vi "index.vi"() -> ()   [LabVIEW 2023]
panel:
  in  "Blank":bool
  in  "label printing":bool
  in  "close call":bool
  in  "Report":bool
  in  "stop":bool
  in  "Vendor Management":bool
  in  "Service Call Entry":bool
  # "Utkarsh Enterprises"
  # "UTKARSH ENTERPRISES"
  # "Developed By- Samarth Wagh (waghsamarth@gmail.com) 7972965098"
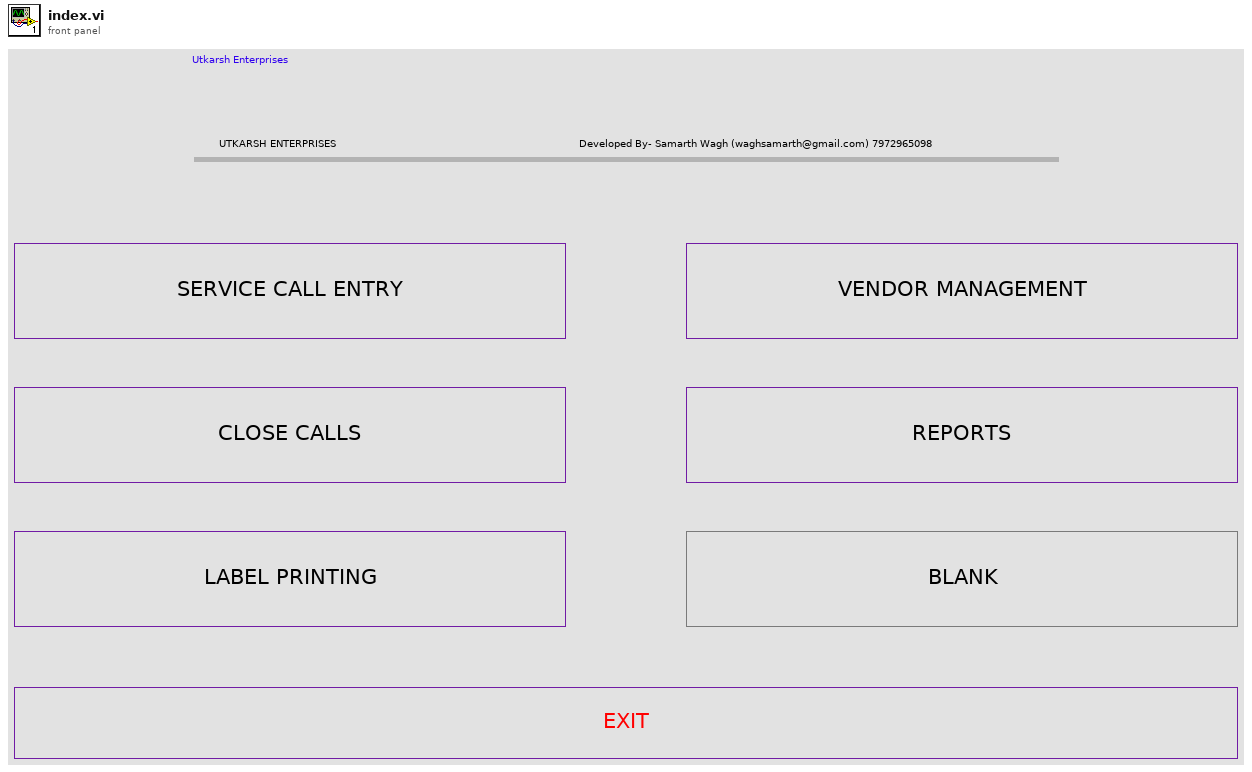
[diagram p1: front panel]
types:
  T1 = enum32{"Invalid", "Standard", "Closed", "Hidden", "Minimized", "Maximized"}
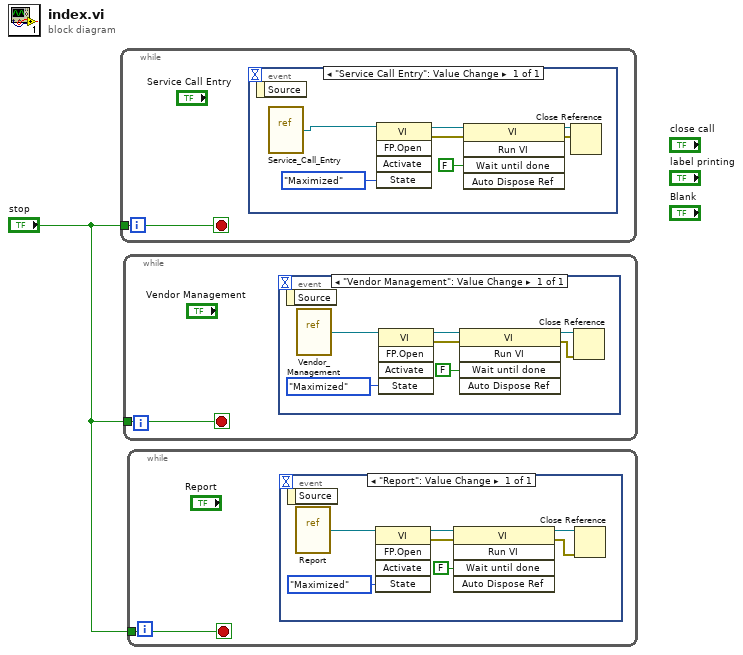
[diagram p0: block diagram]
diagram:
  n1 = while {
    tunnel: "stop" -> [w2]
    stop <- w2 stop-if-true
    n2 = event shown="[0] \"Service Call Entry\": Value Change" {
      selector: _ -> [_]
      dyn-events: _ -> [_]
      timeout: _ -> [_]
      event "Service Call Entry": Value Change {
        n3 = event-data() -> ()  [unwired: 1 in, 1 out]
        n4 = vi-ref "Service_Call_Entry.vi"() -> (w3:refnum<vi>)
        n5 = invoke class="VI" method="FP.Open"(reference=w3, "State"=T1."Maximized") -> (reference out=w9:refnum<vi>, error out=w8:errorcluster)  [unwired: 3 in, 3 out]
        n6 = invoke class="VI" method="Run VI"(reference=w9, error in=w8, "Wait until done"=FALSE) -> (reference out=w4:refnum<vi>, error out=w5:errorcluster)  [unwired: 2 in, 3 out]
        n7 = Close Reference(reference=w4, error in (no error)=w5) -> ()  [unwired: 1 out]
      }
    }
  }
  n8 = while {
    tunnel: "stop" -> [w10]
    stop <- w10 stop-if-true
    n9 = event shown="[0] \"Vendor Management\": Value Change" {
      selector: _ -> [_]
      dyn-events: _ -> [_]
      timeout: _ -> [_]
      event "Vendor Management": Value Change {
        n10 = event-data() -> ()  [unwired: 1 in, 1 out]
        n11 = vi-ref "Vendor_Management.vi"() -> (w17:refnum<vi>)
        n12 = invoke class="VI" method="FP.Open"(reference=w17, "State"=T1."Maximized") -> (reference out=w15:refnum<vi>, error out=w16:errorcluster)  [unwired: 3 in, 3 out]
        n13 = invoke class="VI" method="Run VI"(reference=w15, error in=w16, "Wait until done"=FALSE) -> (reference out=w14:refnum<vi>, error out=w13:errorcluster)  [unwired: 2 in, 3 out]
        n14 = Close Reference(reference=w14, error in (no error)=w13) -> ()  [unwired: 1 out]
      }
    }
  }
  n15 = while {
    tunnel: "stop" -> [w18]
    stop <- w18 stop-if-true
    n16 = event shown="[0] \"Report\": Value Change" {
      selector: _ -> [_]
      dyn-events: _ -> [_]
      timeout: _ -> [_]
      event "Report": Value Change {
        n17 = event-data() -> ()  [unwired: 1 in, 1 out]
        n18 = vi-ref "Report.vi"() -> (w23:refnum<vi>)
        n19 = invoke class="VI" method="FP.Open"(reference=w23, "State"=T1."Maximized") -> (reference out=w21:refnum<vi>, error out=w22:errorcluster)  [unwired: 3 in, 3 out]
        n20 = invoke class="VI" method="Run VI"(reference=w21, error in=w22, "Wait until done"=FALSE) -> (reference out=w24:refnum<vi>, error out=w25:errorcluster)  [unwired: 2 in, 3 out]
        n21 = Close Reference(reference=w24, error in (no error)=w25) -> ()  [unwired: 1 out]
      }
    }
  }
